vi "Read textDecorationRef.vi"(8 "error in (no error)":errorcluster, 11 "TextDecoration in":refnum<class "TextDecoration.lvclass">) -> (0 "error out":errorcluster, 2 "ref":refnum<vi>, 3 "TextDecoration out":refnum<class "TextDecoration.lvclass">)   [LabVIEW 2023, in "TLC_Scripto.lvlib" / "TextDecoration.lvclass"]
uses:
  TextDecoration.lvclass
  C:/projects/TLC_Scripto/Source/GObject/GObject.lvclass
  GObject/Read GObjectRef.vi
  TextDecoration.lvclass/TextDecoration.ctl
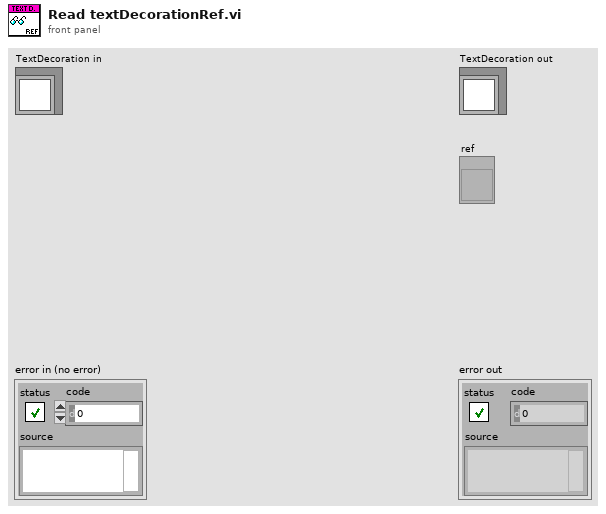
[diagram p1: front panel]
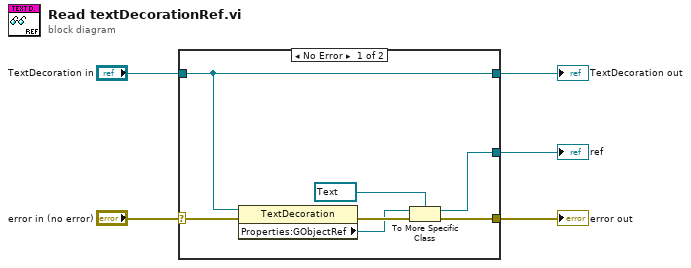
[diagram p0: block diagram]
diagram:
  n1 = case shown="No Error" "error in (no error)" {
    selector: "error in (no error)" -> [w7 w13]
    tunnel: [w6 w13] -> w4
    tunnel: [w12 w14] -> w2
    tunnel: "TextDecoration in" -> [w12 w14]
    tunnel: [w8 _] -> w1
    frame No Error {
      n2 = property class="TextDecoration"(reference=w12, error in=w7) -> (error out=w11:errorcluster, "Properties:GObjectRef"=w10:refnum<vi>)  [unwired: 1 out]
      n3 = To More Specific Class(target class=refnum<vi> refnum ("type"), reference=w10, error in=w11) -> (specific class reference=w8:refnum<vi>, error out=w6:errorcluster)
    }
    frame Error {
    }
  }
  "error out" <- w4
  "TextDecoration out" <- w2
  "ref" <- w1
